vi "MAIN_TL_start_autofocus.vi"(4 "Ref channel":u16(ring) items=["X signal", "Y signal"], 6 "PID gains":T2={"proportional gain (Kc)"=50.0, "integral time (Ti, min)"=0.03, "derivative time (Td, min)"=0.0} {"derivative time (Td, min)" format="%.3f"; "integral time (Ti, min)" format="%.3f"; "proportional gain (Kc)" format="%.3f"}, 7 "queue piezo":refnum<queue>, 8 "error in":errorcluster, 9 "variant":variant, 11 "TL array":dbl[][](array[numeric])) -> (0 "error out":errorcluster, 1 "Next task":T1, 2 "Time lapse  setpoint":dbl, 3 "Channel #":i32)   [LabVIEW 2015]
uses:
  CONTROLS/Q_MCL_piezo_element.ctl
  CONTROLS/Q_main_element.ctl
  GLOBAL/Global_MCL_piezo.vi
  GLOBAL/Global_ABORT.vi
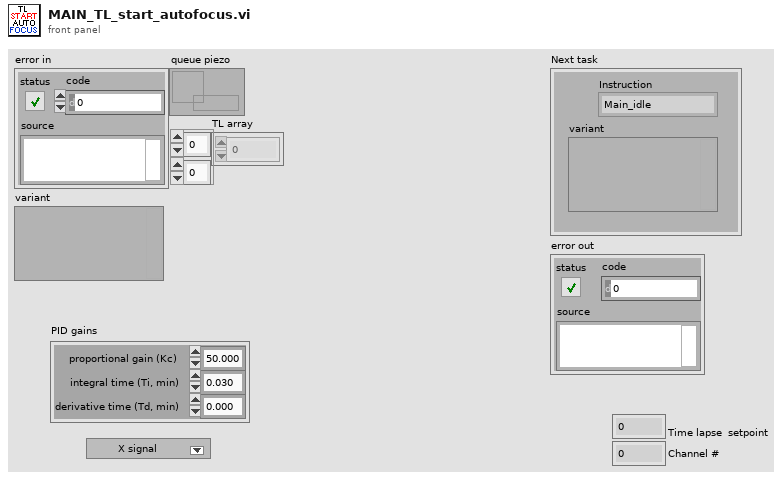
[diagram p1: front panel]
types:
  T1 = typedef "Q_main_element.ctl" = cluster{"variant":variant, "Instruction":enum16{"Main_idle", "Main_initialize", "Main_initialize_TDMS", "Main_initialize_Queue", "Main_error", "Main_DAQ_initialization_results", "Main_ASI_initialization_results", "Main_Piezo_initialization_results", "Main_Valve_initialization_results", "Main_Pump_initialization_results", "Main_CAMERA_initialization_results", "Main_DAQ_error", "Main_ASI_error", "Main_Piezo_error", "Main_CAMERA_error", "Main_Valve_error", "Main_Pump_error", "Main_start_acquiring", "Main_not_acquiring", "Main_acquiring", "Main_stop_acquiring", "Main_change_exposure", "Main_change_z_scan_parameters", "Main_define_ROI", "Main_define_mosaic", "Main_read_kinetic_time", "Main_cooler", "Main_read_temperature", "Main_save_XY", "Main_load_XY", "Main_discard_XY", "Main_move_to_XY", "Main_measure_QPD", "Main_autofocus_calibration", "Main_save_PID", "Main_change_H_valve_position", "Main_two_way_valve", "Main_save_movie", "Main_init_single_scan", "Main_single_scan", "Main_stop_single_scan", "Main_merFISH_illumination_parameters", "Main_merFISH_buffer_probe_list", "Main_merFISH_injections_procedure", "Main_merFISH_save_setpoint", "Main_merFISH_DAPI_parameters", "Main_merFISH_Brightfield_parameters", "Main_merFISH_save_embryo_ROI", "Main_merFISH_init", "Main_merFISH_resume", "Main_merFISH_start_autofocus", "Main_merFISH_open_close_valve_merFISH", "Main_merFISH_open_close_valve_photobleaching", "Main_merFISH_hybridization", "Main_merFISH_move_to_ROI", "Main_merFISH_wait_stabilization", "Main_merFISH_scan_laser", "Main_merFISH_scan_brightfield", "Main_merFISH_photobleaching_injection", "Main_merFISH_photobleaching", "Main_merFISH_save", "Main_merFISH_send_email", "Main_merFISH_close", "Main_TL_define_parameters", "Main_TL_reset_parameters", "Main_TL_init", "Main_TL_start_autofocus", "Main_TL_move_to_ROI", "Main_TL_wait_for_stabilization", "Main_TL_scan", "Main_TL_wait_cycle_end", "Main_TL_close", "Main_STOP"}}
  T2 = cluster{"proportional gain (Kc)":dbl, "integral time (Ti, min)":dbl, "derivative time (Td, min)":dbl}
  T3 = typedef "Q_MCL_piezo_element.ctl" = cluster{"variant":variant, "Instruction":enum16{"Piezo_idle", "Piezo_initialize", "Piezo_error", "Piezo_security_stop", "Piezo_read_z", "Piezo_move_z", "Piezo_keyboard_move", "Piezo_close_autofocus_calibration_ramp", "Piezo_change_init_state", "Piezo_init_autofocus", "Piezo_init_autofocus_merFISH_TL", "Piezo_autofocus", "Piezo_autofocus_merFISH_TL", "Piezo_stop_autofocus", "Piezo_stop_autofocus_merFISH_TL", "Piezo_autofocus_lost", "Piezo_resume_autofocus_merFISH_TL", "Piezo_check_z_position_merFISH_TL", "Piezo_init_ramp", "Piezo_move_z_ramp", "Piezo_close_ramp", "Piezo_close_merFISH", "Piezo_init_TL", "Piezo_close_ramp_TL", "Piezo_close_TL", "Piezo_stop"}}
  T4 = cluster{"PID gains":cluster{"proportional gain (Kc)":dbl, "integral time (Ti, min)":dbl, "derivative time (Td, min)":dbl}, "QPD":cluster{"X":dbl, "Y":dbl, "intensity":dbl}}
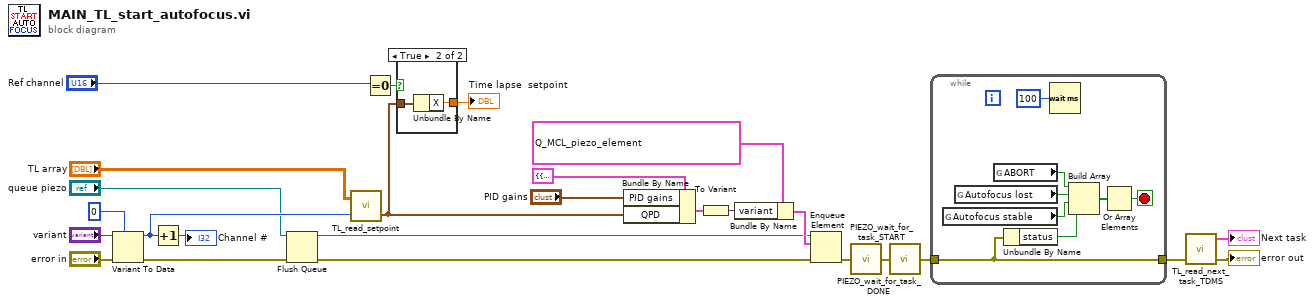
[diagram p0: block diagram]
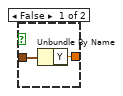
[diagram p2: hidden frame]
diagram:
  n1 = Variant To Data(error in="error in", type=0, Variant="variant") -> (data=w12:i32, error out=w9:errorcluster)
  n2 = Increment(x=w12) -> (x+1=→"Channel #":i32)
  n3 = Flush Queue(queue="queue piezo", error in (no error)=w9) -> (queue out=w16:refnum<queue>, error out=w17:errorcluster)  [unwired: 1 out]
  n4 = call "TL_read_setpoint.vi"("setpoint #"=w12, "TL array"="TL array") -> ("QPD setpoint"=w24:cluster{"X":dbl, "Y":dbl, "intensity":dbl})  [unwired: 1 in]
  n5 = Equal To 0?(x="Ref channel") -> (x = 0?=w23:bool)
  n6 = case shown="True" w23 {
    tunnel: w24 -> [w28 w30]
    tunnel: [w27 w29] -> w25
    frame False {
      n7 = Unbundle By Name(w28) -> ("Y"=w27:dbl)
    }
    frame True {
      n8 = Unbundle By Name(w30) -> ("X"=w29:dbl)
    }
  }
  "Time lapse  setpoint" <- w25
  n9 = Bundle By Name(cluster=T4 {"PID gains"={"proportional gain (Kc)"=2.0, "integral time (Ti, min)"=0.4, "derivative time (Td, min)"=0.0}, "QPD"={"X"=0.0, "Y"=0.0, "intensity"=0.0}}, "PID gains"="PID gains", "QPD"=w24) -> (w14:T4)
  n10 = To Variant(anything=w14) -> (Variant=w15:variant)
  n11 = Bundle By Name(cluster=T3 {"variant"=variant, "Instruction"=enum."Piezo_init_autofocus_merFISH_TL"} ("element"), "variant"=w15) -> (w19:T3)
  n12 = Enqueue Element(queue=w16, element=w19, error in (no error)=w17) -> (error out=w20:errorcluster)  [unwired: 1 in, 2 out]
  n13 = call "PIEZO_wait_for_task_START.vi"("error in"=w20) -> ("error out"=w21:errorcluster)
  n14 = call "PIEZO_wait_for_task_DONE.vi"("error in"=w21) -> ("error out"=w22:errorcluster)
  n15 = while {
    tunnel: [w32] -> w26
    tunnel: w22 -> [w32]
    stop <- w36 stop-if-true
    n16 = global read "Global_MCL_piezo.vi" "Autofocus stable"() -> (w34:bool)
    n17 = global read "Global_MCL_piezo.vi" "Autofocus lost"() -> (w35:bool)
    n18 = global read "Global_ABORT.vi" "ABORT"() -> (w33:bool)
    n19 = Unbundle By Name(w32) -> ("status"=w31:bool)
    n20 = Wait (ms)(milliseconds to wait=u32 100) -> ()  [unwired: 1 out]
    n21 = Build Array(w33, w35, w34, w31) -> (w37:bool[])
    n22 = Or Array Elements(Boolean array=w37) -> (logical OR=w36:bool)
  }
  n23 = call "TL_read_next_task_TDMS.vi"("error in"=w26) -> ("error out"=→"error out":errorcluster, "task"=→"Next task":T1)  [unwired: 3 in]
